vi "test_SessionInitializeErrors_CallCreateSessionsWithInitializeAndDetach_CloseCalledForPreviouslyInitializedSessionsWithProperBehavior.vi"(8 "error in":errorcluster) -> (0 "error out":errorcluster, 2 "result":string, 3 "pass":bool)   [LabVIEW 2020, in "MeasurementServerTests.lvlib"]
uses:
  MeasurementServerTests.lvlib
  Runtime/MeasurementLink Session Management/Session Reservation/Initialize and Close Session Behavior.ctl
  Runtime/MeasurementLink Session Management/Session Reservation/Session Reservation.lvclass
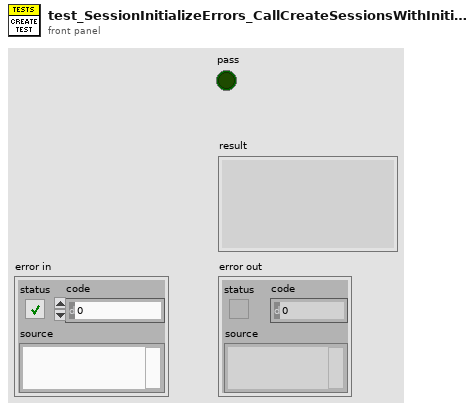
[diagram p1: front panel]
types:
  T1 = typedef "MeasurementLink Session Management.lvlib/Session Reservation.lvclass/Initialize and Close Session Behavior.ctl" = enum16{"Auto", "Initialize and Close", "Attach and Detach", "Initialize and Detach", "Attach and Close"}
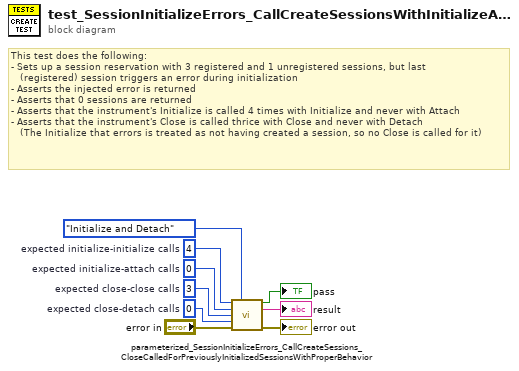
[diagram p0: block diagram]
diagram:
  w5 = u32 0  # expected close-detach calls
  w6 = u32 3  # expected close-close calls
  w7 = u32 0  # expected initialize-attach calls
  w8 = u32 4  # expected initialize-initialize calls
  # "This test does the following:\n- Sets up a session reservation with 3 registered and 1 unregistered sessions, but last\n   (registered) session triggers an error during initialization\n- Asserts the injected error is returned\n- Asserts that 0 sessions are returned\n- Asserts that the instrument's Initialize is called 4 times with Initialize and never with Attach\n- Asserts that the instrument's Close is called thrice with Close and never with Detach\n   (The Initialize that errors is treated as not having created a session, so no Close is called for it)"
  n1 = call "parameterized_SessionInitializeErrors_CallCreateSessions_CloseCalledForPreviouslyInitializedSessionsWithProperBehavior.vi"("expected initialize-initialize calls"=w8, "initialize and close session behavior"=Initialize_and_Close_Session_Behavior."Initialize and Detach", "expected initialize-attach calls"=w7, "expected close-close calls"=w6, "expected close-detach calls"=w5, "error in"="error in") -> ("pass"=→"pass":bool, "result"=→"result":string, "error out"=→"error out":errorcluster)  [unwired: 7 in]
